vi "Connection Info.vi"() -> (2 "Connection Count":i32, 3 "Connected":bool)   [LabVIEW 2017]
doc: "Return basic information about Network Table Connections."
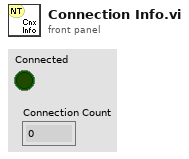
[diagram p1: front panel]
types:
  T1 = enum16{"Add Cnx", "Remove Cnx", "Retrieve List", "Cnx Inited"}
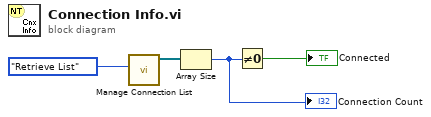
[diagram p0: block diagram]
diagram:
  n1 = call <vilib>:"Manage Connection List.vi"("Operation"=T1."Retrieve List") -> ("Connections List"=w3:refnum<k5>[])  [unwired: 8 in, 2 out]
  n2 = Array Size(array=w3) -> (size(s)=w2:i32)
  "Connection Count" <- w2
  n3 = Not Equal To 0?(x=w2) -> (x != 0?=→"Connected":bool)
